vi "select Platine.vi"(8 "error in":errorcluster, 9 "idListSize":u32, 10 "idList":u32[](array[numeric]), 11 "UI SmarAct in":refnum<class "UI SmarAct.lvclass">) -> (0 "error out":errorcluster, 3 "UI SmarAct out":refnum<class "UI SmarAct.lvclass">)   [LabVIEW 2024, in "UI SmarAct.lvclass"]
doc: "Sélection du controleur MCS smaract"
uses:
  UI SmarAct.lvclass
  UI SmarAct.lvclass/UI SmarAct.ctl
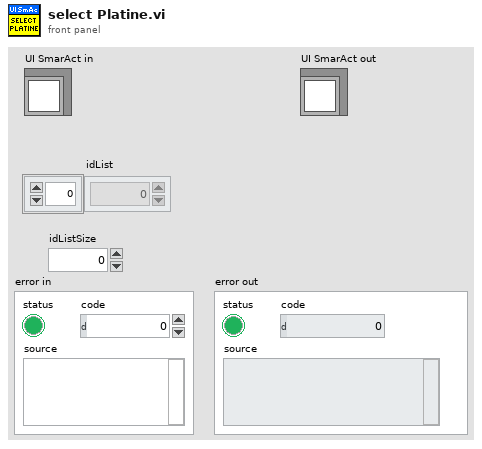
[diagram p1: front panel]
types:
  T1 = enum8{"Enabled", "Disabled", "Disabled and Grayed Out"}
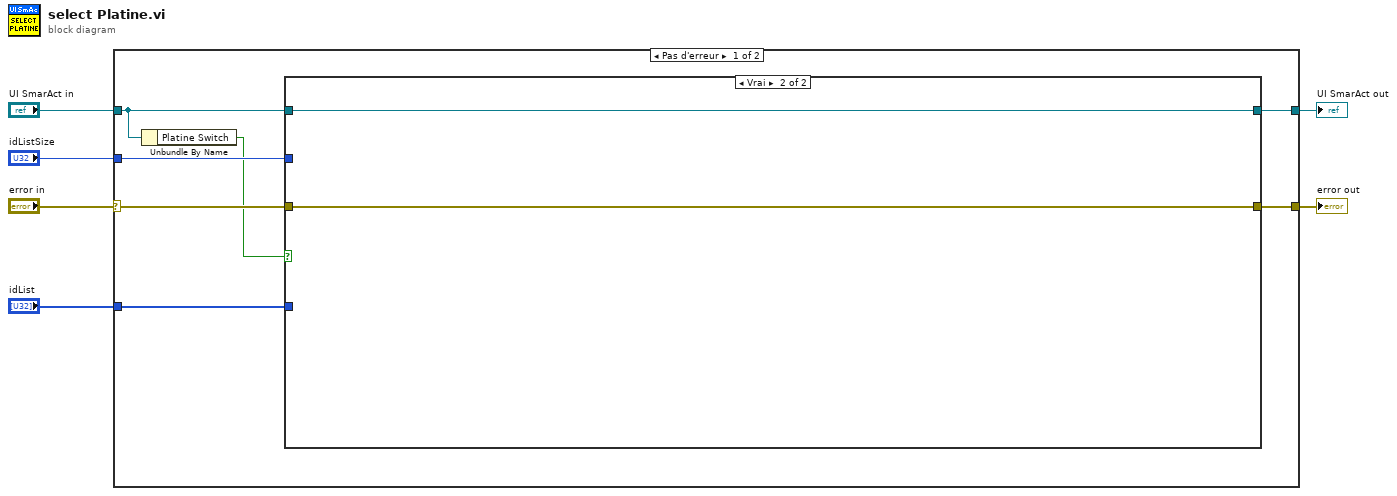
[diagram p0: block diagram]
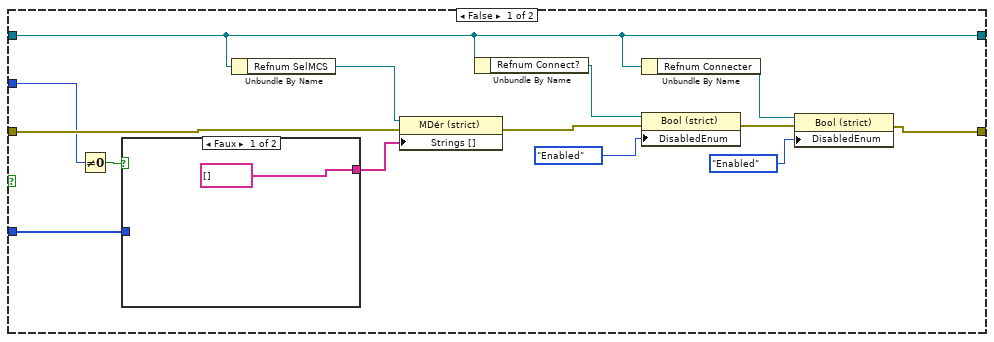
[diagram p2: hidden frame]
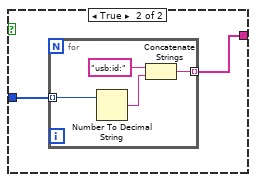
[diagram p3: hidden frame]
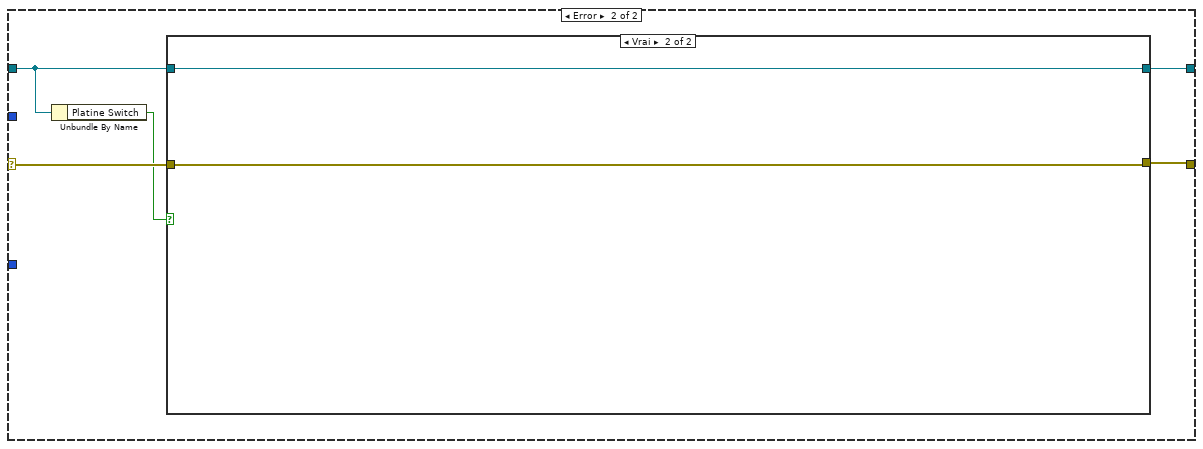
[diagram p4: hidden frame]
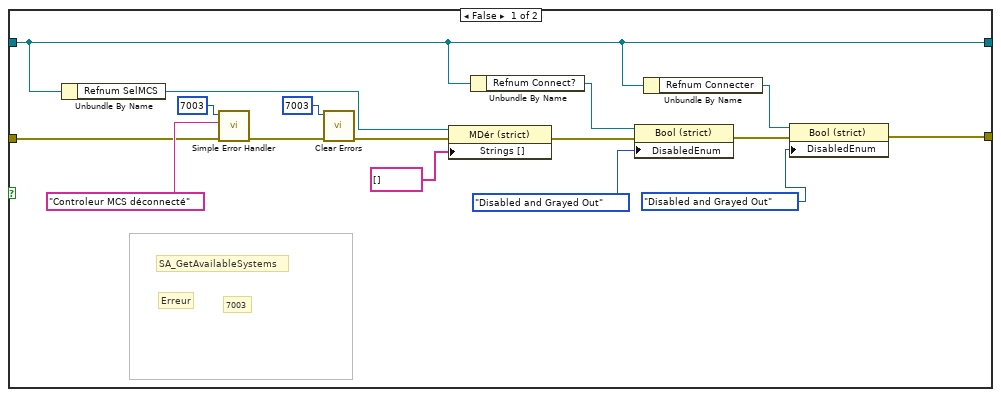
[diagram p5: hidden frame]
diagram:
  n1 = case shown="Pas d'erreur" "error in" {
    selector: "error in" -> [w12 w40]
    tunnel: [w10 w41] -> w6
    tunnel: "idList" -> [w13 _]
    tunnel: "idListSize" -> [w11 _]
    tunnel: "UI SmarAct in" -> [w9 w39]
    tunnel: [w8 w37] -> w2
    frame No Error {
      n2 = Unbundle By Name(w9) -> ("Platine Switch"=w7:bool)
      n3 = case shown="Vrai" w7 {
        tunnel: w13 -> [w26 _]
        tunnel: w12 -> [w25 w35]
        tunnel: w11 -> [w23 _]
        tunnel: [w18 w35] -> w10
        tunnel: w9 -> [w14 w36]
        tunnel: [w14 w36] -> w8
        frame False {
          n4 = Not Equal To 0?(x=w23) -> (x != 0?=w27:bool)
          n5 = case shown="Faux" w27 {
            tunnel: w26 -> [_ w29]
            tunnel: [string[] [] w30] -> w22
            frame False {
            }
            frame True {
              n6 = for {
                tunnel: [w32] -> w30 mode=indexing
                tunnel: w29 -> [w31] mode=indexing
                n7 = Number To Decimal String(number=w31) -> (decimal integer string=w34:string)  [unwired: 1 in]
                n8 = Concatenate Strings("usb:id:", w34) -> (w32:string)
              }
            }
          }
          n9 = Unbundle By Name(w14) -> ("Refnum SelMCS"=w24:refnum<vi>)
          n10 = property class="MDér (strict)"(reference=w24, error in=w25, "Strings []"=w22) -> (error out=w20:errorcluster)  [unwired: 1 out]
          n11 = Unbundle By Name(w14) -> ("Refnum Connect?"=w21:refnum<vi>)
          n12 = Unbundle By Name(w14) -> ("Refnum Connecter"=w17:refnum<vi>)
          n13 = property class="Bool (strict)"(reference=w21, error in=w20, "DisabledEnum"=T1."Enabled" ("Désactivée")) -> (error out=w19:errorcluster)  [unwired: 1 out]
          n14 = property class="Bool (strict)"(reference=w17, error in=w19, "DisabledEnum"=T1."Enabled" ("Désactivée")) -> (error out=w18:errorcluster)  [unwired: 1 out]
        }
        frame True {
        }
      }
    }
    frame Error {
      n15 = Unbundle By Name(w39) -> ("Platine Switch"=w38:bool)
      n16 = case shown="Vrai" w38 {
        tunnel: [w48 w59] -> w41
        tunnel: w39 -> [w42 w58]
        tunnel: w40 -> [w43 w59]
        tunnel: [w42 w58] -> w37
        frame False {
          # "Erreur"
          # "SA_GetAvailableSystems"
          # "7003"
          n17 = Unbundle By Name(w42) -> ("Refnum SelMCS"=w57:refnum<vi>)
          n18 = call <vilib>:"Simple Error Handler.vi"("error code (no error:0)"=7003, "error source (\" \")"="Controleur MCS déconnecté" ("error source (\" \")"), "error in (no error)"=w43) -> ("error out"=w56:errorcluster)  [unwired: 2 in, 4 out]
          n19 = call <vilib>:"Clear Errors.vi"("error in (no error)"=w56, "specific error code to clear (0: all)"=7003) -> ("error out"=w55:errorcluster)  [unwired: 4 in, 1 out]
          n20 = property class="MDér (strict)"(reference=w57, error in=w55, "Strings []"=string[] []) -> (error out=w49:errorcluster)  [unwired: 1 out]
          n21 = Unbundle By Name(w42) -> ("Refnum Connect?"=w46:refnum<vi>)
          n22 = property class="Bool (strict)"(reference=w46, error in=w49, "DisabledEnum"=T1."Disabled and Grayed Out" ("Désactivée")) -> (error out=w50:errorcluster)  [unwired: 1 out]
          n23 = Unbundle By Name(w42) -> ("Refnum Connecter"=w47:refnum<vi>)
          n24 = property class="Bool (strict)"(reference=w47, error in=w50, "DisabledEnum"=T1."Disabled and Grayed Out" ("Désactivée")) -> (error out=w48:errorcluster)  [unwired: 1 out]
        }
        frame True {
        }
      }
    }
  }
  "error out" <- w6
  "UI SmarAct out" <- w2
